vi "Handler - Next Step.vi"(8 "error in (no error)":errorcluster, 11 "RT - Analysis Data in":T1={"RTController Data"={"State"=enum."Idle", "APU Setup Info"={"[[Sensor Info]]"=[], "[[Calibration Info]]"=[], "[[CMM Table 106]]"=[], "[[General APU Info]]"=[], "General APU Information"={"Run Count"=0}}, "Testing Select"=enum."Manual", "APU Select"="<Select>", "Subtests Array"=[], "Current Subtest&Step Indices"=[], "Fuel Pressure Regulator"=4.0, "Bleed-Fuel-ECS Controls"={"Bleed-Coarse-Knob"=0.0, "Bleed-Coarse-RapidClose"=FALSE, "Bleed-Coarse-RapidOpen"=FALSE, "Bleed-Coarse-Frozen"=FALSE, "Bleed-Fine-Knob"=0.0, "Bleed-Fine-RapidClose"=FALSE, "Bleed-Fine-RapidOpen"=FALSE, "Bleed-Fine-Frozen"=FALSE}, "ECS Demand Cluster"={"02.06.9265.02"=4.0}, "APU & ECU Controls"={"02.00.9485.00"=FALSE, "02.01.9485.03"=FALSE, "02.01.9485.00"=FALSE, "02.01.9485.01"=FALSE, "02.00.9485.01"=FALSE, "02.00.9485.02"=FALSE, "02.00.9485.03"=FALSE, "02.00.9485.04"=FALSE, "02.00.9485.05"=FALSE, "02.01.9485.06"=FALSE, "02.00.9485.07"=FALSE, "00.04.9265.03"=FALSE}}, "Analyzed Data Sets"=[], "Current Vals"={"Post-Analysis Data"={"Calibrated Data"={"00-00-9205 Calib"=[], "00-01-9205 Calib"=[], "01-00-9213 Calib"=[], "01-01-9213 Calib"=[], "01-02-9213 Calib"=[], "02-02-9219 Calib"=[], "02-03-9227 Calib"=[], "00-02-9234 Calib"=[], "00-03-9402 Calib"=[], "02-05-9205 Calib"=[], "02-04-9871 2DArray"=[]}, "Calculated Data"={"C.00"=0.0, "C.01"=0.0, "C.02"=0.0, "C.03"=0.0, "C.04"=0.0, "C.05"=0.0, "C.06"=0.0, "C.07"=0.0, "C.08"=0.0, "C.09"=0.0, "C.10"=0.0, "C.11"=0.0, "C.12"=0.0, "C.13"=0.0, "C.14"=0.0, "C.15"=0.0, "C.16"=0.0, "C.17"=0.0, "C.18"=0.0, "C.19"=0.0, "C.20"=0.0, "C.21"=0.0, "C.22"=0.0, "C.23"=0.0, "C.24"=0.0, "C.25"=0.0, "C.26"=0.0, "C.27"=0.0, "C.28"=0.0, "C.29"=0.0, "C.30"=0.0, "C.31"=0.0, "C.32"=0.0, "C.33"=0.0, "C.34"=0.0, "C.35"=0.0, "C.36"=0.0, "C.37"=0.0, "C.38"=0.0, "C.39"=0.0, "C.40"=0.0, "C.41"=0.0, "C.42"=0.0, "C.43"=0.0, "C.44"=0.0, "C.45"=0.0, "C.46"=0.0, "C.47"=0.0, "C.48"=0.0, "C.49"=0.0, "C.50"=0.0, "C.51"=0.0, "C.52"=0.0, "C.53"=0.0, "C.54"=0.0, "C.56"=0.0}, "Indicator Data"={"00-02-9234 Power Spectras"=[], "00-02-9234 Peak Vel (in/sec)"=[], "Interactive Mode Vals"=[]}}, "Parsed Data Arrays"={"[Parsed Tags]"=[], "[VData out]"=[], "[Whole Tags]"=[]}}, "Samples/Sec"=0.0, "User Input Vals"=[], "Watchdogs"=[], "Interactive Data"={"Confirm Pressed"=FALSE, "Stored Vals"=[]}} {"RTController Data"."ECS Demand Cluster"."02.06.9265.02" min=0.0 max=10.0 step=0.25 scale=0.0..10.0; "RTController Data"."Bleed-Fuel-ECS Controls"."Bleed-Fine-Knob" min=0.0 max=1.0 step=0.001 scale=0.0..1.0; "RTController Data"."Bleed-Fuel-ECS Controls"."Bleed-Coarse-Knob" min=0.0 max=1.0 step=0.001 scale=0.0..1.0; "RTController Data"."Fuel Pressure Regulator" min=0.0 max=100.0 step=0.25 scale=4.0..20.0}) -> (0 "error out":errorcluster, 3 "RT - Analysis Data out":T1={"RTController Data"={"State"=enum."Idle", "APU Setup Info"={"[[Sensor Info]]"=[], "[[Calibration Info]]"=[], "[[CMM Table 106]]"=[], "[[General APU Info]]"=[], "General APU Information"={"Run Count"=0}}, "Testing Select"=enum."Manual", "APU Select"="<Select>", "Subtests Array"=[], "Current Subtest&Step Indices"=[], "Fuel Pressure Regulator"=4.0, "Bleed-Fuel-ECS Controls"={"Bleed-Coarse-Knob"=0.0, "Bleed-Coarse-RapidClose"=FALSE, "Bleed-Coarse-RapidOpen"=FALSE, "Bleed-Coarse-Frozen"=FALSE, "Bleed-Fine-Knob"=0.0, "Bleed-Fine-RapidClose"=FALSE, "Bleed-Fine-RapidOpen"=FALSE, "Bleed-Fine-Frozen"=FALSE}, "ECS Demand Cluster"={"02.06.9265.02"=4.0}, "APU & ECU Controls"={"02.00.9485.00"=FALSE, "02.01.9485.03"=FALSE, "02.01.9485.00"=FALSE, "02.01.9485.01"=FALSE, "02.00.9485.01"=FALSE, "02.00.9485.02"=FALSE, "02.00.9485.03"=FALSE, "02.00.9485.04"=FALSE, "02.00.9485.05"=FALSE, "02.01.9485.06"=FALSE, "02.00.9485.07"=FALSE, "00.04.9265.03"=FALSE}}, "Analyzed Data Sets"=[], "Current Vals"={"Post-Analysis Data"={"Calibrated Data"={"00-00-9205 Calib"=[], "00-01-9205 Calib"=[], "01-00-9213 Calib"=[], "01-01-9213 Calib"=[], "01-02-9213 Calib"=[], "02-02-9219 Calib"=[], "02-03-9227 Calib"=[], "00-02-9234 Calib"=[], "00-03-9402 Calib"=[], "02-05-9205 Calib"=[], "02-04-9871 2DArray"=[]}, "Calculated Data"={"C.00"=0.0, "C.01"=0.0, "C.02"=0.0, "C.03"=0.0, "C.04"=0.0, "C.05"=0.0, "C.06"=0.0, "C.07"=0.0, "C.08"=0.0, "C.09"=0.0, "C.10"=0.0, "C.11"=0.0, "C.12"=0.0, "C.13"=0.0, "C.14"=0.0, "C.15"=0.0, "C.16"=0.0, "C.17"=0.0, "C.18"=0.0, "C.19"=0.0, "C.20"=0.0, "C.21"=0.0, "C.22"=0.0, "C.23"=0.0, "C.24"=0.0, "C.25"=0.0, "C.26"=0.0, "C.27"=0.0, "C.28"=0.0, "C.29"=0.0, "C.30"=0.0, "C.31"=0.0, "C.32"=0.0, "C.33"=0.0, "C.34"=0.0, "C.35"=0.0, "C.36"=0.0, "C.37"=0.0, "C.38"=0.0, "C.39"=0.0, "C.40"=0.0, "C.41"=0.0, "C.42"=0.0, "C.43"=0.0, "C.44"=0.0, "C.45"=0.0, "C.46"=0.0, "C.47"=0.0, "C.48"=0.0, "C.49"=0.0, "C.50"=0.0, "C.51"=0.0, "C.52"=0.0, "C.53"=0.0, "C.54"=0.0, "C.56"=0.0}, "Indicator Data"={"00-02-9234 Power Spectras"=[], "00-02-9234 Peak Vel (in/sec)"=[], "Interactive Mode Vals"=[]}}, "Parsed Data Arrays"={"[Parsed Tags]"=[], "[VData out]"=[], "[Whole Tags]"=[]}}, "Samples/Sec"=0.0, "User Input Vals"=[], "Watchdogs"=[], "Interactive Data"={"Confirm Pressed"=FALSE, "Stored Vals"=[]}} {"RTController Data"."ECS Demand Cluster"."02.06.9265.02" min=0.0 max=10.0 step=0.25 scale=0.0..10.0; "RTController Data"."Bleed-Fuel-ECS Controls"."Bleed-Fine-Knob" min=0.0 max=1.0 step=0.001 scale=0.0..1.0; "RTController Data"."Bleed-Fuel-ECS Controls"."Bleed-Coarse-Knob" min=0.0 max=1.0 step=0.001 scale=0.0..1.0; "RTController Data"."Fuel Pressure Regulator" min=0.0 max=100.0 step=0.25 scale=4.0..20.0})   [LabVIEW 2014]
uses:
  RT - Host Comms/RT - Host Comms.lvlib
  Modules/cRIO RT Comms/Private Controls/Stream Data.ctl
  Modules/cRIO RT Comms/cRIO RT Comms.lvlib
  Top Level/Shared Controls/cRIO State.ctl
  Modules/Controller (Host)/Public Controls/Testing Select.ctl
  Modules/Controller (Host)/Controller (Host).lvlib
  Modules/Controller (Host)/Public Controls/APU Select.ctl
  Private Controls/RTController Data.ctl
  RT - Analysis.lvlib
  Private Controls/RT-Analysis Data.ctl
  Top Level/Shared Controls/Acq Data.ctl
  Top Level/Shared Controls/Post-Analysis Data.ctl
  Top Level/Shared Controls/Analyzed Data Sets.ctl
  Modules/Testing UI 1/Public Controls/Fuel Pressure Regulator.ctl
  Modules/Testing UI 1/Testing UI 1.lvlib
  Modules/Testing UI 1/Public Controls/Bleed-Fuel-ECS Controls.ctl
  Modules/Testing UI 1/Public Controls/ECS Demand Controls.ctl
  Modules/Testing UI 1/Private Controls/APU & ECU Controls.ctl
  Top Level/Shared Controls/APU Setup File.ctl
  Top Level/Shared Controls/Calculated Data.ctl
  Top Level/Shared Controls/All Data Cluster.ctl
  Modules/File IO/Public Controls/General APU Info.ctl
  Modules/File IO/File IO.lvlib
  Top Level/Shared Controls/Parsed Tag Cluster.ctl
  Private Controls/Parsed Data Arrays.ctl
  Private Controls/Watchdog Settings.ctl
  Private Controls/Interactive Data.ctl
panel:
  # "GTCP331-200ER Control Panel Discrete Input Panel"
  # "Bleed Load Controls"
  # "GTCP331-200ER Control Panel Discrete Input Panel"
  # "Bleed Load Controls"
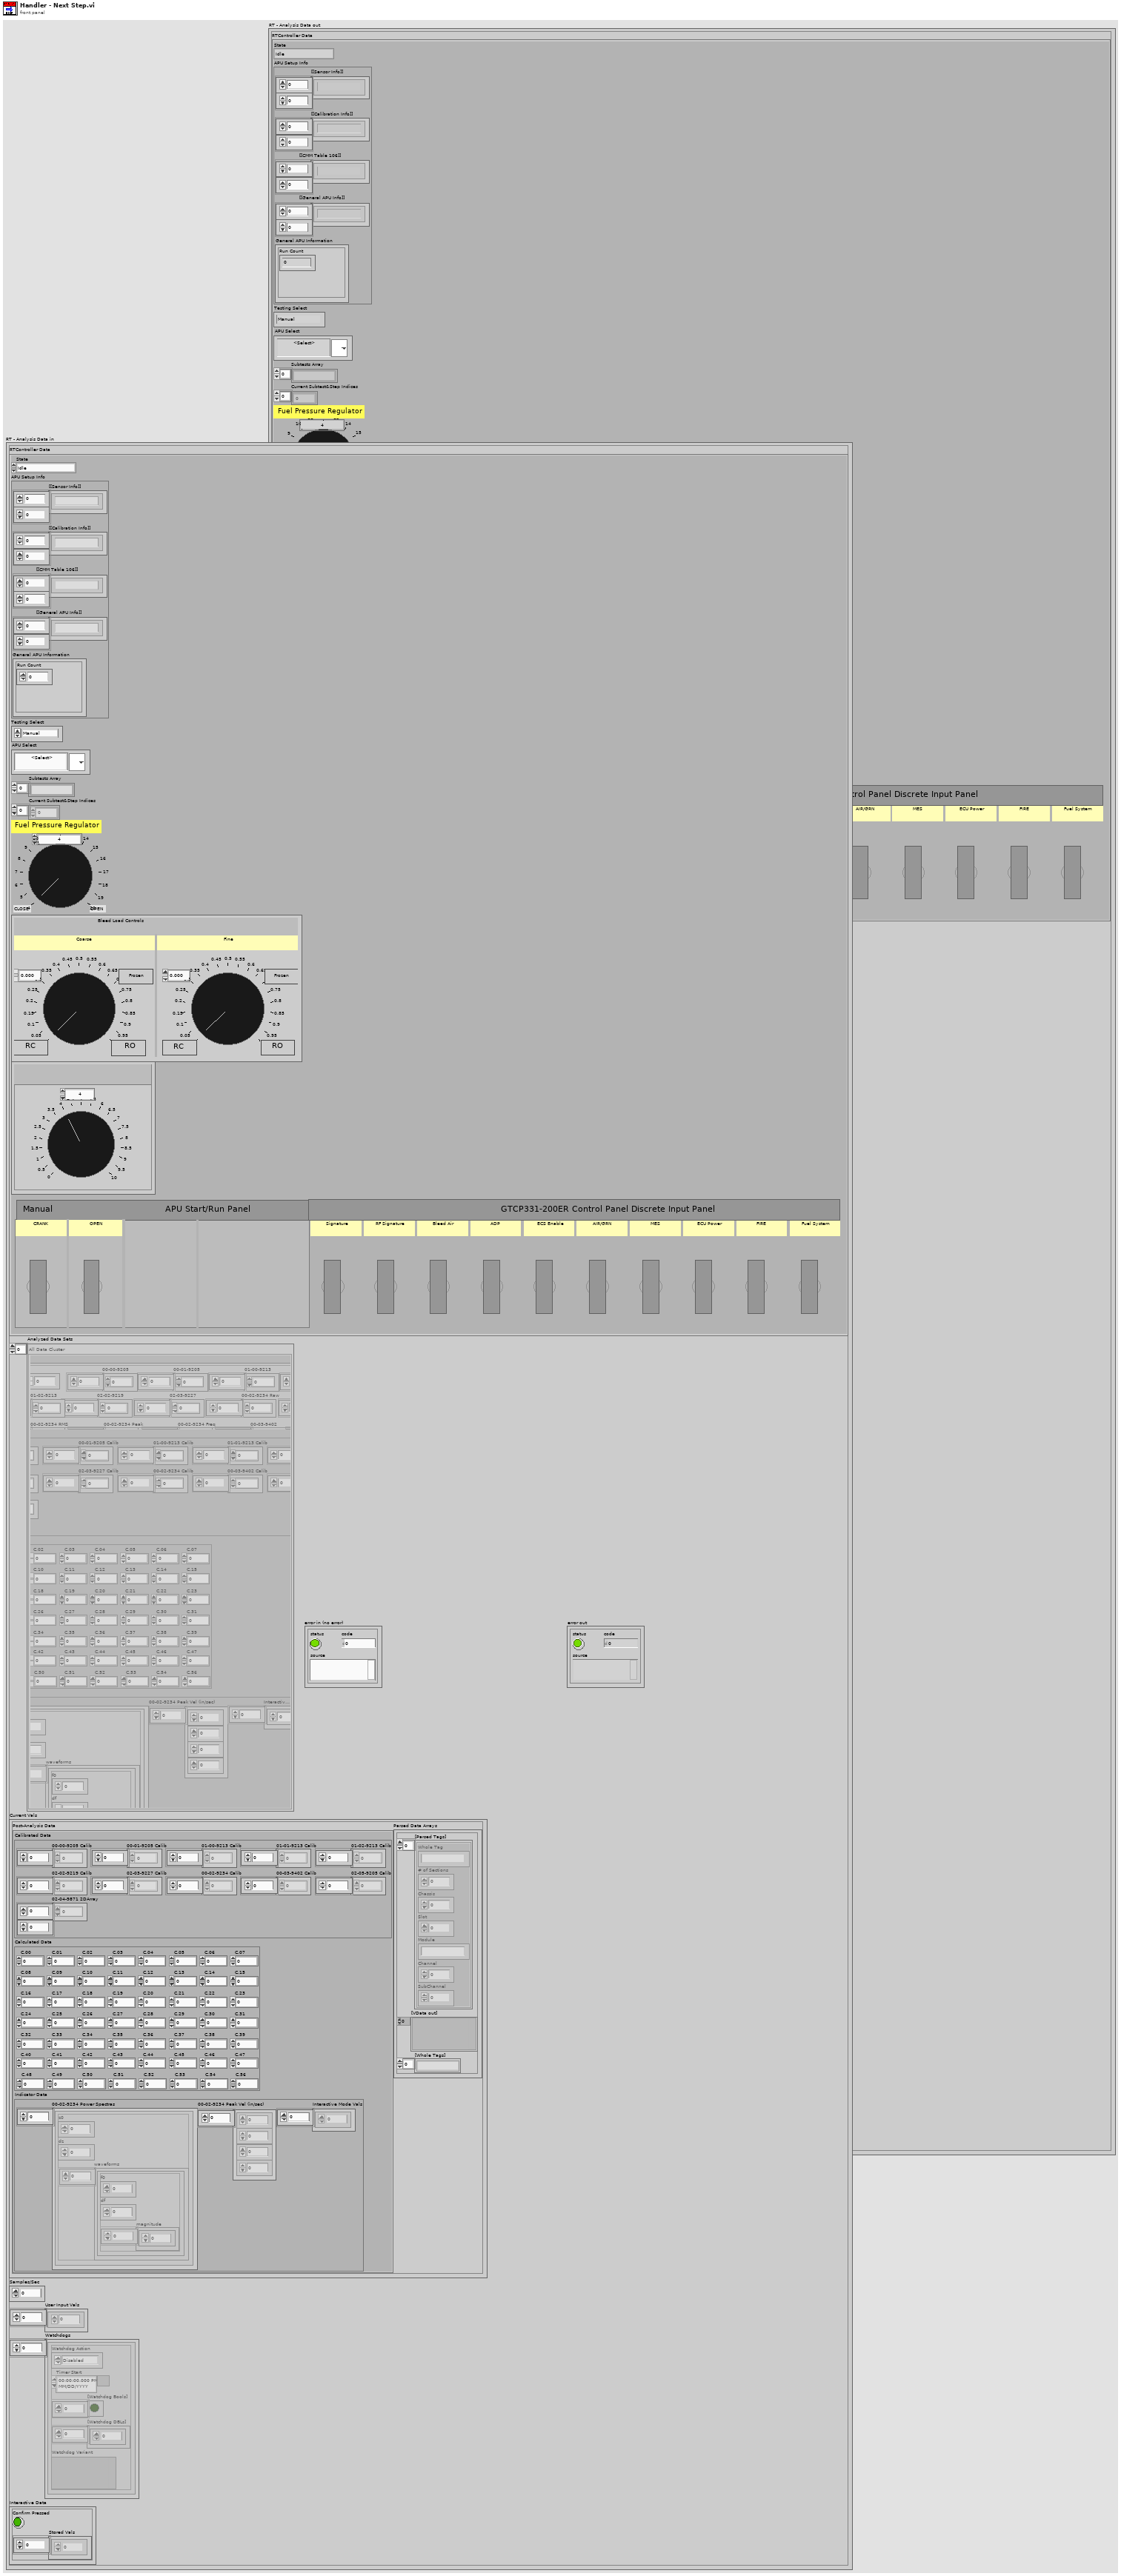
[diagram p1: front panel]
types:
  T1 = typedef "RT - Analysis.lvlib/RT-Analysis Data.ctl" = cluster{"RTController Data":T2, "Analyzed Data Sets":T12, "Current Vals":cluster{"Post-Analysis Data":T15, "Parsed Data Arrays":T17}, "Samples/Sec":dbl, "User Input Vals":dbl[], "Watchdogs":T19[], "Interactive Data":T20}
  T2 = typedef "RT - Analysis.lvlib/RTController Data.ctl" = cluster{"State":T3, "APU Setup Info":T4, "Testing Select":T6, "APU Select":T7, "Subtests Array":string[], "Current Subtest&Step Indices":i32[], "Fuel Pressure Regulator":T8, "Bleed-Fuel-ECS Controls":T9, "ECS Demand Cluster":T10, "APU & ECU Controls":T11}
  T3 = typedef "cRIO State.ctl" = enum16{"Waiting for Cal Info", "Idle", "Calibration", "Testing"}
  T4 = typedef "APU Setup File.ctl" = cluster{"[[Sensor Info]]":string[][], "[[Calibration Info]]":string[][], "[[CMM Table 106]]":string[][], "[[General APU Info]]":string[][], "General APU Information":T5}
  T5 = typedef "File IO.lvlib/General APU Info.ctl" = cluster{"Run Count":u64}
  T6 = typedef "Controller (Host).lvlib/Testing Select.ctl" = enum16{"Manual", "Interactive", "Automatic"}
  T7 = typedef "Controller (Host).lvlib/APU Select.ctl" = string
  T8 = typedef "Testing UI 1.lvlib/Fuel Pressure Regulator.ctl" = dbl
  T9 = typedef "Testing UI 1.lvlib/Bleed-Fuel-ECS Controls.ctl" = cluster{"Bleed-Coarse-Knob":dbl, "Bleed-Coarse-RapidClose":bool, "Bleed-Coarse-RapidOpen":bool, "Bleed-Coarse-Frozen":bool, "Bleed-Fine-Knob":dbl, "Bleed-Fine-RapidClose":bool, "Bleed-Fine-RapidOpen":bool, "Bleed-Fine-Frozen":bool}
  T10 = typedef "Testing UI 1.lvlib/ECS Demand Controls.ctl" = cluster{"02.06.9265.02":dbl}
  T11 = typedef "Testing UI 1.lvlib/APU & ECU Controls.ctl" = cluster{"02.00.9485.00":bool, "02.01.9485.03":bool, "02.01.9485.00":bool, "02.01.9485.01":bool, "02.00.9485.01":bool, "02.00.9485.02":bool, "02.00.9485.03":bool, "02.00.9485.04":bool, "02.00.9485.05":bool, "02.01.9485.06":bool, "02.00.9485.07":bool, "00.04.9265.03":bool}
  T12 = typedef "Analyzed Data Sets.ctl" = T13[]
  T13 = typedef "All Data Cluster.ctl" = cluster{"Acq Data":T14, "Post-Analysis Data":T15}
  T14 = typedef "Acq Data.ctl" = cluster{"Timestamp":timestamp, "Acq Period (ms)":i64, "00-00-9205":dbl[], "00-01-9205":dbl[], "01-00-9213":dbl[], "01-01-9213":dbl[], "01-02-9213":dbl[], "02-02-9219":dbl[], "02-03-9227":dbl[], "00-02-9234 Raw":dbl[], "00-02-9234 DC":dbl[], "00-02-9234 RMS":dbl[], "00-02-9234 Peak":dbl[], "00-02-9234 Freq":dbl[], "00-03-9402":dbl[], "02-05-9205":dbl[], "02-04-9871":dbl[]}
  T15 = typedef "Post-Analysis Data.ctl" = cluster{"Calibrated Data":cluster{"00-00-9205 Calib":dbl[], "00-01-9205 Calib":dbl[], "01-00-9213 Calib":dbl[], "01-01-9213 Calib":dbl[], "01-02-9213 Calib":dbl[], "02-02-9219 Calib":dbl[], "02-03-9227 Calib":dbl[], "00-02-9234 Calib":dbl[], "00-03-9402 Calib":dbl[], "02-05-9205 Calib":dbl[], "02-04-9871 2DArray":dbl[][]}, "Calculated Data":T16, "Indicator Data":cluster{"00-02-9234 Power Spectras":cluster{"z0":dbl, "dz":dbl, "waveforms":cluster{"f0":dbl, "df":dbl, "magnitude":dbl[]}[]}[], "00-02-9234 Peak Vel (in/sec)":dbl[], "Interactive Mode Vals":dbl[]}}
  T16 = typedef "Calculated Data.ctl" = cluster{"C.00":dbl, "C.01":dbl, "C.02":dbl, "C.03":dbl, "C.04":dbl, "C.05":dbl, "C.06":dbl, "C.07":dbl, "C.08":dbl, "C.09":dbl, "C.10":dbl, "C.11":dbl, "C.12":dbl, "C.13":dbl, "C.14":dbl, "C.15":dbl, "C.16":dbl, "C.17":dbl, "C.18":dbl, "C.19":dbl, "C.20":dbl, "C.21":dbl, "C.22":dbl, "C.23":dbl, "C.24":dbl, "C.25":dbl, "C.26":dbl, "C.27":dbl, "C.28":dbl, "C.29":dbl, "C.30":dbl, "C.31":dbl, "C.32":dbl, "C.33":dbl, "C.34":dbl, "C.35":dbl, "C.36":dbl, "C.37":dbl, "C.38":dbl, "C.39":dbl, "C.40":dbl, "C.41":dbl, "C.42":dbl, "C.43":dbl, "C.44":dbl, "C.45":dbl, "C.46":dbl, "C.47":dbl, "C.48":dbl, "C.49":dbl, "C.50":dbl, "C.51":dbl, "C.52":dbl, "C.53":dbl, "C.54":dbl, "C.56":dbl}
  T17 = typedef "RT - Analysis.lvlib/Parsed Data Arrays.ctl" = cluster{"[Parsed Tags]":T18[], "[VData out]":variant[], "[Whole Tags]":string[]}
  T18 = typedef "Parsed Tag Cluster.ctl" = cluster{"Whole Tag":string, "# of Sections":u8, "Chassis":u8, "Slot":u8, "Module":string, "Channel":u8, "SubChannel":u8}
  T19 = typedef "RT - Analysis.lvlib/Watchdog Settings.ctl" = cluster{"Watchdog Action":enum16{"Disabled", "Timer - Change Sample Rate", "RPM Thresh - Insert Other", "RPM Thresh - Check POPD", "RPM Thresh - StartStop Logging"}, "Timer Start":timestamp, "[Watchdog Bools]":bool[], "[Watchdog DBLs]":dbl[], "Watchdog Variant":variant}
  T20 = typedef "RT - Analysis.lvlib/Interactive Data.ctl" = cluster{"Confirm Pressed":bool, "Stored Vals":dbl[]}
  T21 = typedef "cRIO RT Comms.lvlib/Stream Data.ctl" = cluster{"Action":string, "Data":variant}
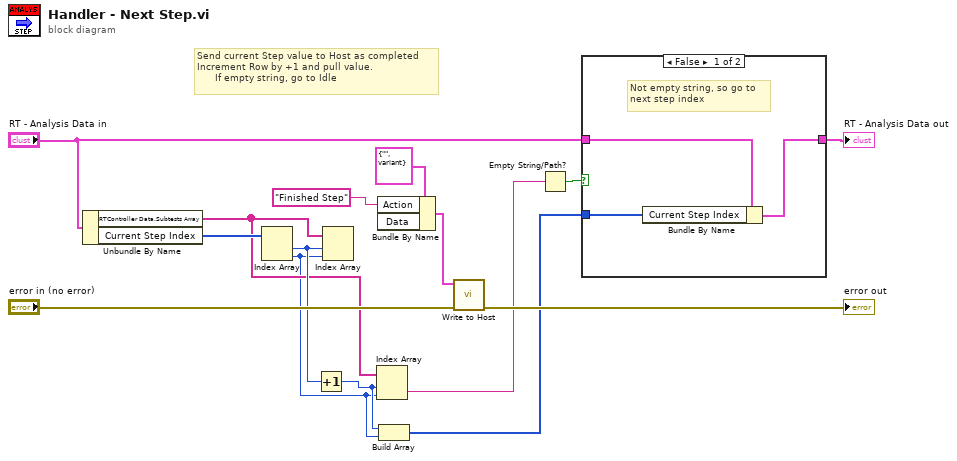
[diagram p0: block diagram]
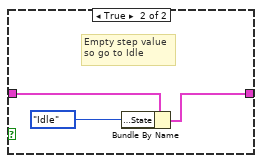
[diagram p2: hidden frame]
diagram:
  # "Send current Step value to Host as completed\nIncrement Row by +1 and pull value.\n      If empty string, go to Idle"
  n1 = Unbundle By Name("RT - Analysis Data in") -> ("RTController Data.Subtests Array"=w5:string[], "Current Step Index"=w6:i32[])
  n2 = Index Array(array=w6) -> (element #1=w8:i32, element #2=w3:i32)  [unwired: 2 in]
  n3 = Increment(x=w8) -> (x+1=w4:i32)
  n4 = Index Array(array=w5, index (row)=w8, index (col)=w3) -> ()  [unwired: 1 out]
  n5 = Index Array(array=w5, index (row)=w4, index (col)=w3) -> (element=w7:string)
  n6 = Bundle By Name(cluster=T21 {"Action"="", "Data"=variant} ("data in"), "Action"="Finished Step") -> (w10:T21)  [unwired: 1 in]
  n7 = Build Array(w4, w3) -> (w2:i32[])
  n8 = call "Write to Host.vi"("error in (no error)"="error in (no error)", "data in"=w10) -> ("error out"=→"error out":errorcluster)  [unwired: 9 in]
  n9 = Empty String/Path?(string/path=w7) -> (empty?=w1:bool)
  n10 = case shown="False" w1 {
    tunnel: [w17 w20] -> w15
    tunnel: "RT - Analysis Data in" -> [w18 w21]
    tunnel: w2 -> [w16 _]
    frame False {
      # "Not empty string, so go to\nnext step index"
      n11 = Bundle By Name(cluster=w18, "Current Step Index"=w16) -> (w17:T1)
    }
    frame True {
      # "Empty step value\nso go to Idle"
      n12 = Bundle By Name(cluster=w21, "RTController Data.State"=cRIO_State."Idle") -> (w20:T1)
    }
  }
  "RT - Analysis Data out" <- w15
